vi "Agilent 34970 Multifunction.vi"() -> ()   [LabVIEW 2016]
doc: "This VI shows how to use the HP34907A module. It gives examples of using the DAC, totalizer, and digital in/out channels."
uses:
  Agilent 34970.lvlib
panel:
  in  "Serial Port Configuration":T1={"Timeout Value (10000)"=10000, "Baud Rate (57600)"=enum."57600", "Flow Control (1:XON/XOFF)"=enum."XON / XOFF"}
  in  "Reset":bool=TRUE
  in  "VISA resource name":refnum<visa-resource-name>
  in  "Slot Number":u8=1 min=1 max=3 step=1
  out "Digital Value Read":bool[](array[boolean])
  in  "Digital Value Write (0)":bool[](array[boolean])=[FALSE, FALSE, FALSE, FALSE, FALSE, FALSE, FALSE, FALSE, FALSE, FALSE, FALSE, FALSE, FALSE, FALSE, FALSE, FALSE]
  out "Totalalizer\nCount":u32
  in  "Function":T2(ring)
  in  "Voltage":dbl(knob) min=-12.0 max=12.0 step=0.001 scale=-12.0..12.0 scale format="%.2f"
  in  "Channel":bool
  # "(c) 2005-2010 National Instruments.  ALL RIGHTS RESERVED."
  # "Using the \"Slot Number\" control, choose the slot in the HP34970A containing the multifunction \nmodule (HP34907A).  Next choose what you want to write or read using the \"Function\" control.\n\nThe \"Channel\" control chooses which channel to use with the Send Analog, Read Digital, and\nWrite Digital functions."
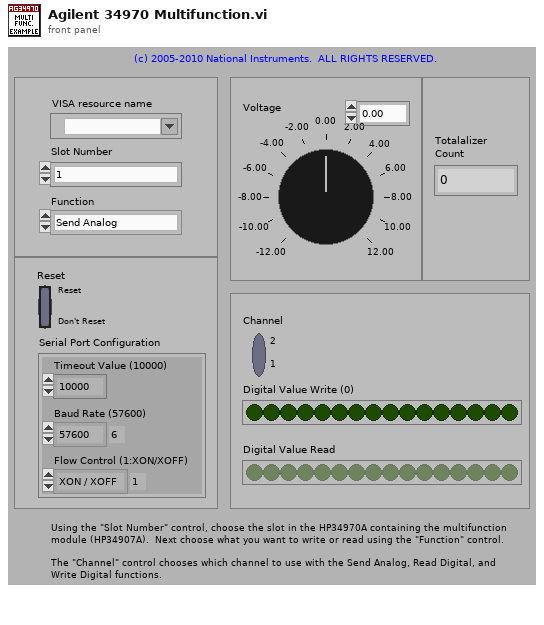
[diagram p1: front panel]
types:
  T1 = cluster{"Timeout Value (10000)":u32, "Baud Rate (57600)":enum16{"1200", "2400", "4800", "9600", "19200", "38400", "57600", "115200"}, "Flow Control (1:XON/XOFF)":enum16{"None", "XON / XOFF", "RTS / CTS", "DTR / DSR"}}
  T2 = enum16{"Send Analog", "Send Digital", "Read Totalizer", "Read Word", "Read Byte"}
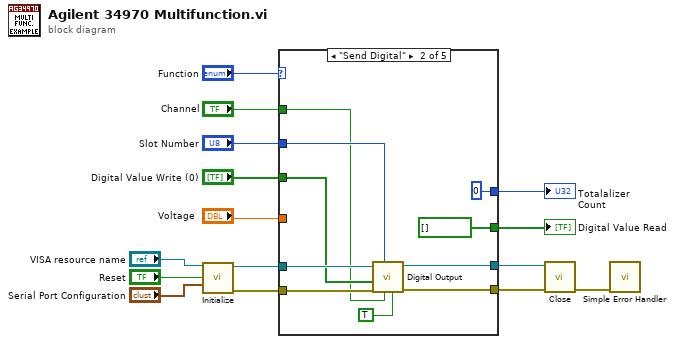
[diagram p0: block diagram]
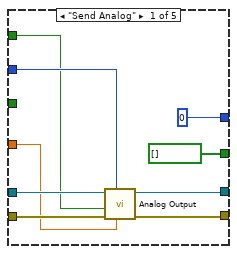
[diagram p2: hidden frame]
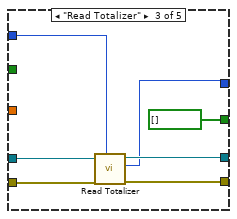
[diagram p3: hidden frame]
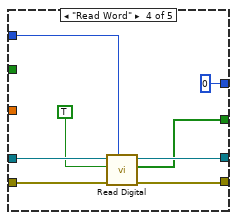
[diagram p4: hidden frame]
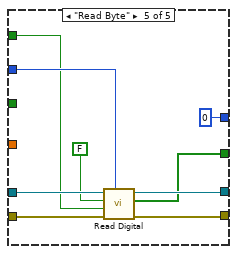
[diagram p5: hidden frame]
diagram:
  n1 = call "Initialize.vi"("VISA Resource Name"="VISA resource name", "Reset (T: Reset)"="Reset", "Serial Port Configuration"="Serial Port Configuration") -> ("VISA Resource Name Out"=w9:refnum<visa-resource-name>, "error out"=w8:errorcluster)  [unwired: 11 in]
  n2 = case shown="\"Send Digital\"" "Function" {
    tunnel: "Channel" -> [w16 w25 _ _ w50]
    tunnel: w8 -> [w22 w30 w40 w47 w57]
    tunnel: w9 -> [w23 w33 w41 w48 w58]
    tunnel: [u32 0 u32 0 w36 u32 0 u32 0 ("Total")] -> w14
    tunnel: "Voltage" -> [w18 _ _ _ _]
    tunnel: "Slot Number" -> [w19 w29 w39 w44 w54]
    tunnel: [w21 w32 w38 w46 w56] -> w7
    tunnel: [w20 w31 w37 w45 w55] -> w6
    tunnel: "Digital Value Write (0)" -> [_ w28 _ _ _]
    tunnel: [bool[] [] ("Digital Value") bool[] [] ("Digital Value") bool[] [] ("Digital Value") w42 w52] -> w13
    frame "Send Analog" {
      n3 = call "Analog Output.vi"("Voltage (0)"=w18, "Slot Number (1)"=w19, "error in (no error)"=w22, "Analog Output (F:1)"=w16, "VISA Resource Name"=w23) -> ("error out"=w20:errorcluster, "VISA Resource Name Out"=w21:refnum<visa-resource-name>)  [unwired: 4 in, 1 out]
    }
    frame "Send Digital" {
      n4 = call "Digital Output.vi"("Check Byte/Word (F:Byte)"=TRUE, "Check Digital Port (F:Port 1)"=w25, "Slot Number (1)"=w29, "error in (no error)"=w30, "DIO Write (All F:0)"=w28, "VISA Resource Name"=w33) -> ("error out"=w31:errorcluster, "VISA Resource Name Out"=w32:refnum<visa-resource-name>)  [unwired: 3 in, 1 out]
    }
    frame "Read Totalizer" {
      n5 = call "Read Totalizer.vi"("Slot Number (1)"=w39, "error in (no error)"=w40, "VISA Resource Name"=w41) -> ("error out"=w37:errorcluster, "Total"=w36:u32, "VISA Resource Name Out"=w38:refnum<visa-resource-name>)  [unwired: 6 in]
    }
    frame "Read Word" {
      n6 = call "Read Digital.vi"("Slot Number (1)"=w44, "error in (no error)"=w47, "Byte/Word (F:Byte)"=TRUE, "VISA Resource Name"=w48) -> ("error out"=w45:errorcluster, "Digital Value"=w42:bool[], "VISA Resource Name Out"=w46:refnum<visa-resource-name>)  [unwired: 5 in]
    }
    frame "Read Byte" {
      n7 = call "Read Digital.vi"("Slot Number (1)"=w54, "error in (no error)"=w57, "Digital Port (F:1)"=w50, "Byte/Word (F:Byte)"=FALSE, "VISA Resource Name"=w58) -> ("error out"=w55:errorcluster, "Digital Value"=w52:bool[], "VISA Resource Name Out"=w56:refnum<visa-resource-name>)  [unwired: 4 in]
    }
  }
  "Totalalizer\nCount" <- w14
  "Digital Value Read" <- w13
  n8 = call "Close.vi"("VISA Resource Name"=w7, "error in (no error)"=w6) -> ("error out"=w5:errorcluster)  [unwired: 13 in]
  n9 = call <vilib>:"Simple Error Handler.vi"("error in (no error)"=w5) -> ()  [unwired: 4 in, 5 out]
